vi "Get HTTPS Port.vi"(8 "error in (no error)":errorcluster, 11 "Server in":refnum<class "Server.lvclass">) -> (0 "error out":errorcluster, 2 "HTTPS Port":u16, 3 "Server out":refnum<class "Server.lvclass">)   [LabVIEW 2020, in "HTTP Server.lvlib" / "Server.lvclass"]
uses:
  Server.lvclass
  Server.lvclass/Server.ctl
  lv-uri/URI/URI/URI.lvclass
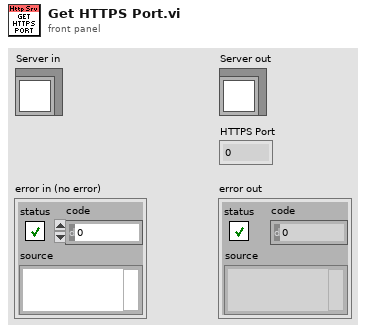
[diagram p1: front panel]
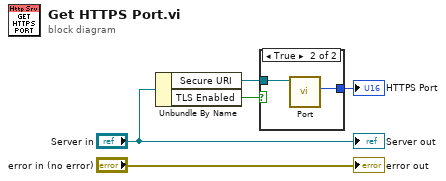
[diagram p0: block diagram]
diagram:
  n1 = Unbundle By Name("Server in") -> ("Secure URI"=w2:refnum<class "URI.lvclass">, "TLS Enabled"=w3:bool)
  n2 = case shown="True" w3 {
    tunnel: w2 -> [_ w6]
    tunnel: [_ w7] -> w1
    frame False {
    }
    frame True {
      n3 = call "Port.vi"("URI in"=w6) -> ("Port"=w7:u16)  [unwired: 8 in, 2 out]
    }
  }
  "HTTPS Port" <- w1
  "error out" <- "error in (no error)"
  "Server out" <- "Server in"
